vi "LakeShore350.vi"() -> ()   [LabVIEW 2015]
uses:
  SECoP.lvlib
  <vilib>/regexp/Match Regular Expression.xnode
  Program Files (x86)/National Instruments/LabVIEW 2016/instr.lib/Lake Shore 350/Lake Shore 350.lvlib
  parametertype.ctl
panel:
  out "error out":errorcluster
  out "log":string
  in  "DLL path":path=path "C:/Users/user/Desktop/x86_32"
  in  "stop":bool
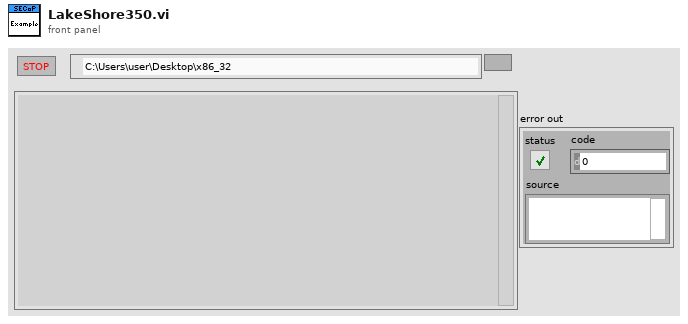
[diagram p1: front panel]
types:
  T1 = typedef "parametertype.ctl" = enum8{"readonly", "readwrite", "command"}
  T2 = cluster{"name":string, "type":T1, "datatype":string, "description":string}[]
  T3 = cluster{"Baud Rate":u32, "Parity":u16, "Data Bits":u16, "Stop Bits":u16, "Flow Control":u16}
  T4 = typedef "SECoP.lvlib/SECoP-libraries.ctl" = cluster{"serverDLL":path, "variantDLL":path, "cleanup_mode":bool}
  T5 = typedef "SECoP.lvlib/SECoP-action.ctl" = enum32{"any action", "read", "change", "do cmd"}
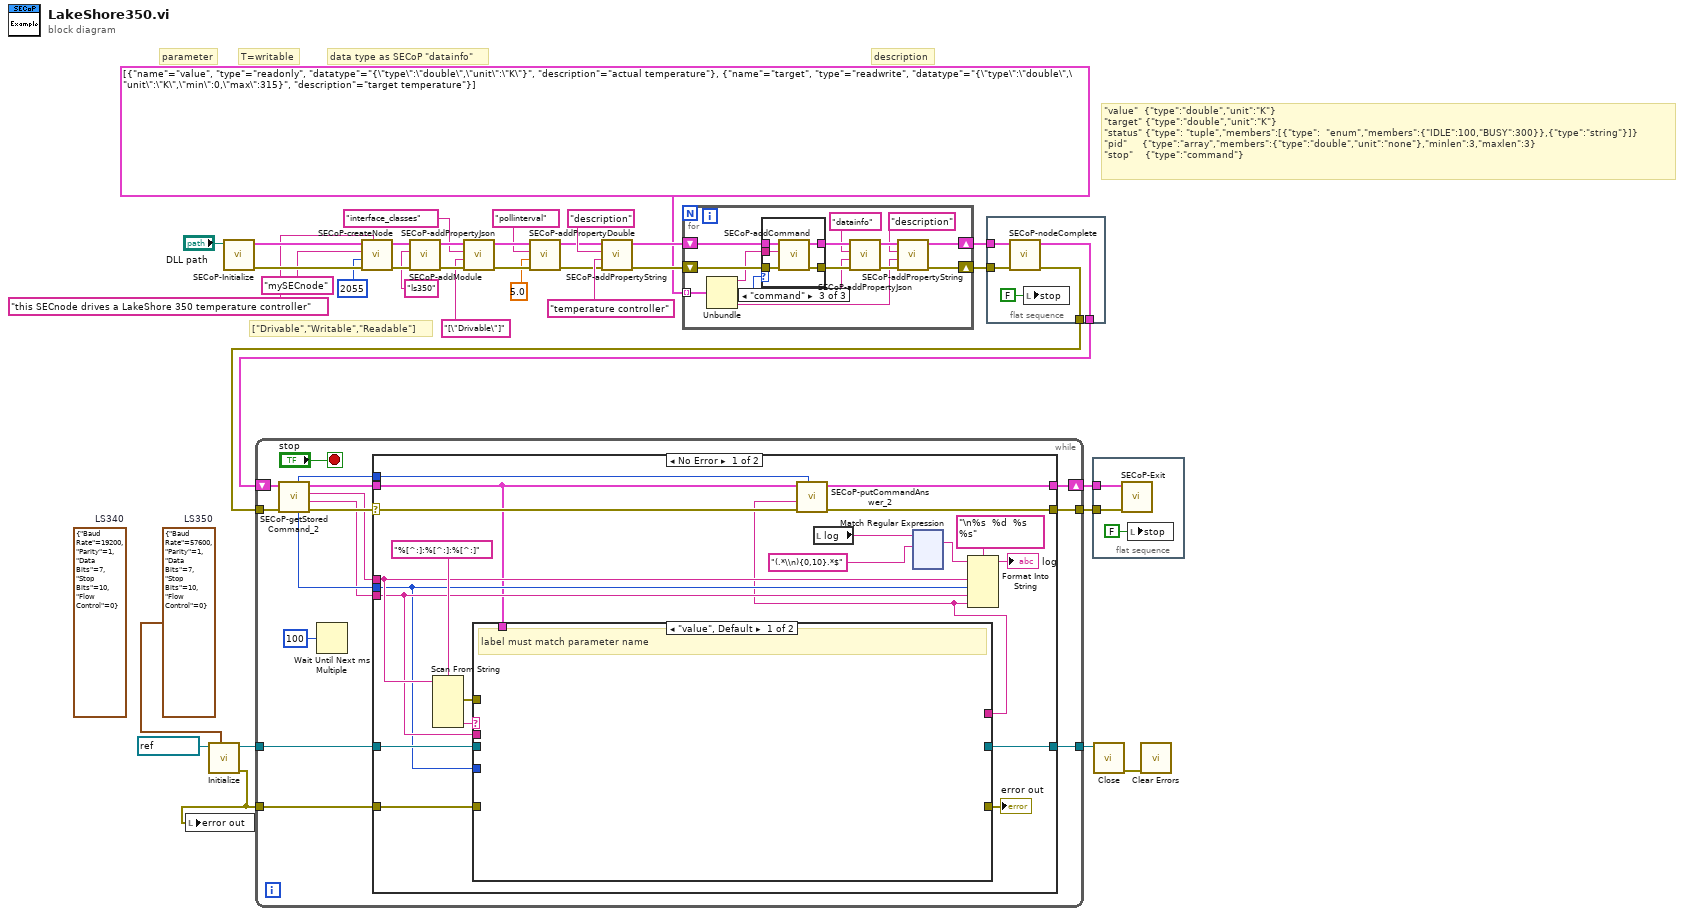
[diagram p0: block diagram]
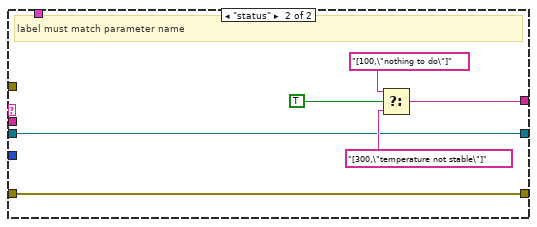
[diagram p2: hidden frame]
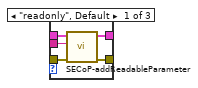
[diagram p4: hidden frame]
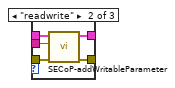
[diagram p5: hidden frame]
diagram:
  (unwired) T3 {"Baud Rate"=19200, "Parity"=1, "Data Bits"=7, "Stop Bits"=10, "Flow Control"=0}  # LS340
  w2 = T3 {"Baud Rate"=57600, "Parity"=1, "Data Bits"=7, "Stop Bits"=10, "Flow Control"=0}  # LS350
  # "description"
  # "data type as SECoP \"datainfo\""
  # "T=writable"
  # "parameter"
  # "[\"Drivable\",\"Writable\",\"Readable\"]"
  # "\"value\"  {\"type\":\"double\",\"unit\":\"K\"}\n\"target\" {\"type\":\"double\",\"unit\":\"K\"}\n\"status\" {\"type\": \"tuple\",\"members\":[{\"type\":  \"enum\",\"members\":{\"IDLE\":100,\"BUSY\":300}},{\"type\":\"string\"}]}\n\"pid\"     {\"type\":\"array\",\"members\":{\"type\":\"double\",\"unit\":\"none\"},\"minlen\":3,\"maxlen\":3}\n\"stop\"    {\"type\":\"command\"}"
  n1 = call "Initialize.vi"("Serial Configuration"=w2, "VISA resource name"=refnum<visa-resource-name> "COM4") -> ("error out"=w3:errorcluster, "VISA resource name out"=w6:refnum<visa-resource-name>)  [unwired: 8 in]
  n2 = local write "error out"(w3) -> ()
  n3 = call "SECoP-Initialize.vi"("DLL path (in)"="DLL path") -> ("error out"=w34:errorcluster, "DLL path (out)"=w35:T4)  [unwired: 9 in]
  n4 = while {
    shift-right: [w51] -> w23
    shift-left: w10 -> [w49]
    tunnel: w11 -> [w48]
    tunnel: [w41] -> w22
    tunnel: w6 -> [w39]
    tunnel: [w38] -> w5
    tunnel: w3 -> [w37]
    stop <- "stop" stop-if-true
    n5 = call "SECoP-getStoredCommand_2.vi"("error in (no error)"=w48, "DLL path (in)"=w49) -> ("error out"=w46:errorcluster, "arguments/setvalue"=w42:string, "command/parameter path"=w43:string, "DLL path (out)"=w47:T4, "action"=w44:T5, "command id"=w45:u64)  [unwired: 4 in]
    n6 = Wait Until Next ms Multiple(millisecond multiple=u32 100) -> ()  [unwired: 1 out]
    n7 = case shown="No Error" w46 {
      selector: w46 -> [w72 w194]
      tunnel: w47 -> [w52 w195]
      tunnel: [w71 w195] -> w51
      tunnel: w45 -> [w70 _]
      tunnel: w43 -> [w63 _]
      tunnel: w42 -> [w58 _]
      tunnel: w44 -> [w57 _]
      tunnel: [w69 w194] -> w41
      tunnel: w39 -> [w59 w193]
      tunnel: [w56 w193] -> w38
      tunnel: w37 -> [w54 _]
      frame No Error {
        n8 = Scan From String(format string="%[^:]:%[^:]:%[^:]", input string=w63) -> (error out=w61:errorcluster, output 3=w62:string)  [unwired: 7 in, 2 out]
        n9 = case shown="\"value\", Default" w62 {
          tunnel: [_ w76] -> w53
          tunnel: w61 -> [_ _]
          tunnel: w59 -> [_ w74]
          tunnel: w58 -> [_ _]
          tunnel: [_ w74] -> w56
          tunnel: w57 -> [_ _]
          tunnel: [_ w75] -> w55
          tunnel: w54 -> [_ w75]
          tunnel: w52 -> [_ _]
          frame "value", Default {
            # "label must match parameter name"
          }
          frame "status" {
            # "label must match parameter name"
            n10 = Select(t="[100,\"nothing to do\"]", s=TRUE, f="[300,\"temperature not stable\"]") -> (s? t:f=w76:string)
          }
        }
        "error out" <- w55
        n11 = call "SECoP-putCommandAnswer_2.vi"("command id"=w70, "error in (no error)"=w72, "value"=w53, "DLL path (in)"=w52) -> ("error out"=w69:errorcluster, "DLL path (out)"=w71:T4)  [unwired: 6 in]
        n12 = local read "log"() -> (w66:string)
        n13 = xnode "Match Regular Expression"("input string"=w66, "regular expression"="(.*\\n){0,10}.*$") -> ("whole match"=w67:string)  [unwired: 4 in, 4 out]
        n14 = Format Into String(format string="\n%s  %d  %s  %s", initial string=w67, w63, w57, w58, w53) -> (resulting string=→"log":string)  [unwired: 1 in, 1 out]
      }
      frame Error {
      }
    }
  }
  n15 = call "SECoP-createNode.vi"("description"="this SECnode drives a LakeShore 350 temperature controller", "error in (no error)"=w34, "TCP port"=u16 2055, "node id"="mySECnode" ("id"), "DLL path (in)"=w35) -> ("error out"=w29:errorcluster, "DLL path (out)"=w33:T4)  [unwired: 5 in]
  n16 = call "SECoP-addModule.vi"("error in (no error)"=w29, "module name"="ls350" ("name"), "DLL path (in)"=w33) -> ("error out"=w26:errorcluster, "DLL path (out)"=w27:T4)  [unwired: 7 in]
  n17 = call "SECoP-addPropertyJson.vi"("error in (no error)"=w26, "property value"="[\"Drivable\"]" ("name"), "property name"="interface_classes" ("name"), "DLL path (in)"=w27) -> ("error out"=w15:errorcluster, "DLL path (out)"=w17:T4)  [unwired: 6 in]
  n18 = call "SECoP-addPropertyDouble.vi"("error in (no error)"=w15, "property value"=5.0, "property name"="pollinterval", "DLL path (in)"=w17) -> ("error out"=w14:errorcluster, "DLL path (out)"=w16:T4)  [unwired: 6 in]
  n19 = call "SECoP-addPropertyString.vi"("error in (no error)"=w14, "property value"="temperature controller" ("name"), "property name"="description" ("name"), "DLL path (in)"=w16) -> ("error out"=w20:errorcluster, "DLL path (out)"=w21:T4)  [unwired: 6 in]
  n20 = for {
    tunnel: T2 [{"name"="value", "type"=enum."readonly", "datatype"="{\"type\":\"double\",\"unit\":\"K\"}", "description"="actual temperature"}, {"name"="target", "type"=enum."readwrite", "datatype"="{\"type\":\"double\",\"unit\":\"K\",\"min\":0,\"max\":315}", "description"="target temperature"}] -> [w198] mode=indexing
    shift-right: [w197] -> w9
    shift-left: w21 -> [w207]
    shift-right: [w196] -> w8
    shift-left: w20 -> [w206]
    n21 = Unbundle(w198) -> ("name"=w199:string, "type"=w208:T1, "datatype"=w200:string, "description"=w201:string)
    n22 = case shown="\"command\"" w208 {
      tunnel: w199 -> [w213 w220 w221]
      tunnel: w207 -> [w215 w219 w225]
      tunnel: [w214 w218 w222] -> w205
      tunnel: [w211 w216 w223] -> w204
      tunnel: w206 -> [w212 w217 w224]
      frame "readonly", Default {
        n23 = call "SECoP-addReadableParameter.vi"("error in (no error)"=w212, "parameter name"=w213, "DLL path (in)"=w215) -> ("error out"=w211:errorcluster, "DLL path (out)"=w214:T4)  [unwired: 7 in]
      }
      frame "readwrite" {
        n24 = call "SECoP-addWritableParameter.vi"("error in (no error)"=w217, "parameter name"=w220, "DLL path (in)"=w219) -> ("error out"=w216:errorcluster, "DLL path (out)"=w218:T4)  [unwired: 7 in]
      }
      frame "command" {
        n25 = call "SECoP-addCommand.vi"("error in (no error)"=w224, "command name"=w221, "DLL path (in)"=w225) -> ("error out"=w223:errorcluster, "DLL path (out)"=w222:T4)  [unwired: 7 in]
      }
    }
    n26 = call "SECoP-addPropertyJson.vi"("error in (no error)"=w204, "property value"=w200, "property name"="datainfo" ("name"), "DLL path (in)"=w205) -> ("error out"=w209:errorcluster, "DLL path (out)"=w210:T4)  [unwired: 6 in]
    n27 = call "SECoP-addPropertyString.vi"("error in (no error)"=w209, "property value"=w201, "property name"="description" ("name"), "DLL path (in)"=w210) -> ("error out"=w196:errorcluster, "DLL path (out)"=w197:T4)  [unwired: 6 in]
  }
  n28 = flat-sequence {
    tunnel: w9 -> [w229]
    tunnel: w8 -> [w228]
    tunnel: [w226] -> w10
    tunnel: [w227] -> w11
    frame #0 {
      n29 = call "SECoP-nodeComplete.vi"("error in (no error)"=w228, "DLL path (in)"=w229) -> ("error out"=w227:errorcluster, "DLL path (out)"=w226:T4)  [unwired: 8 in]
      n30 = local write "stop"(FALSE) -> ()
    }
  }
  n31 = flat-sequence {
    tunnel: w23 -> [w232]
    tunnel: w22 -> [w231]
    frame #0 {
      n32 = call "SECoP-Exit.vi"("error in (no error)"=w231, "DLL path (in)"=w232) -> ()  [unwired: 9 in, 1 out]
      n33 = local write "stop"(FALSE) -> ()
    }
  }
  n34 = call "Close.vi"("VISA resource name"=w5) -> ("error out"=w4:errorcluster)  [unwired: 10 in]
  n35 = call <vilib>:"Clear Errors.vi"("error in (no error)"=w4) -> ()  [unwired: 5 in, 2 out]
